vi "Check_Create Folder.vi"(8 "error in (no error)":errorcluster, 10 "Folder Name":string, 11 "Base Path":path) -> (0 "error out":errorcluster, 3 "Folder Path":path)   [LabVIEW 2010, in "lib1299.lvlib"]
uses:
  lib1299.lvlib
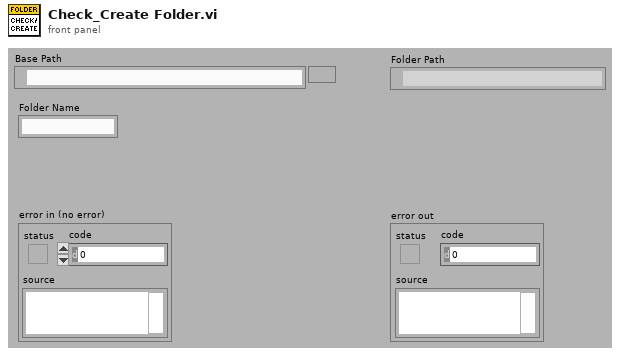
[diagram p1: front panel]
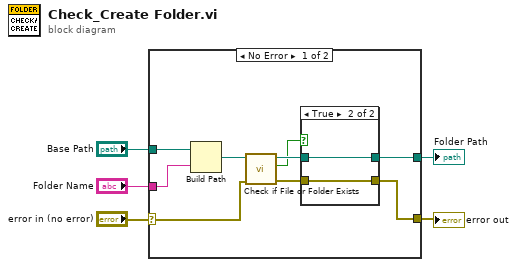
[diagram p0: block diagram]
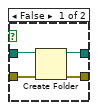
[diagram p2: hidden frame]
diagram:
  n1 = case shown="No Error" "error in (no error)" {
    selector: "error in (no error)" -> [w6 w22]
    tunnel: [w13 w22] -> w5
    tunnel: [w11 w21] -> w4
    tunnel: "Folder Name" -> [w8 _]
    tunnel: "Base Path" -> [w7 w21]
    frame No Error {
      n2 = Build Path(base path=w7, name or relative path=w8) -> (appended path=w9:path)
      n3 = call <vilib>:"Check if File or Folder Exists.vi"("error in (no error)"=w6, "path"=w9) -> ("error out"=w14:errorcluster, "file or folder exists?"=w10:bool, "dup path"=w12:path)  [unwired: 7 out]
      n4 = case shown="True" w10 {
        tunnel: [w17 w20] -> w11
        tunnel: w12 -> [w18 w20]
        tunnel: [w16 w19] -> w13
        tunnel: w14 -> [w15 w19]
        frame False {
          n5 = Create Folder(path (use dialog)=w18, error in=w15) -> (created path=w17:path, error out=w16:errorcluster)  [unwired: 2 out]
        }
        frame True {
        }
      }
    }
    frame Error {
    }
  }
  "error out" <- w5
  "Folder Path" <- w4
